vi "Re-Sample Waveform (SubVI).vi"(9 "Filtered w/f":dbl[](array[numeric]), 10 "old dt":dbl, 11 "Re Sample Rate(Hz)":dbl=1000.0 format="%#_13g") -> (2 "Re-sampled w/f":dbl[](array[numeric]), 3 "new dt":dbl)   [LabVIEW 2017]
uses:
  <vilib>/measure/NI_MAPro.lvlib
  <vilib>/measure/maresamp.llb/Resample Waveform (single shot).vi
panel:
  out "error out":errorcluster
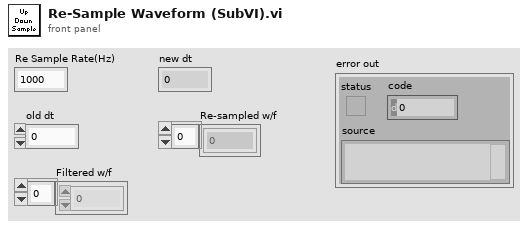
[diagram p1: front panel]
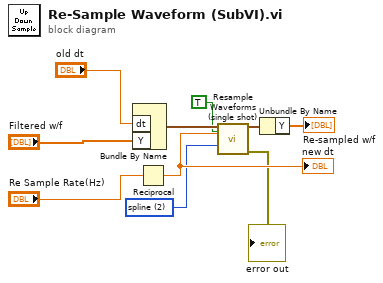
[diagram p0: block diagram]
diagram:
  w4 = u16 2 items=["coerce", "linear", "spline", "FIR filter"] ("interpolation mode")
  n1 = Bundle By Name("dt"="old dt", "Y"="Filtered w/f") -> (w5:waveform(dbl))  [unwired: 1 in]
  n2 = Reciprocal(x="Re Sample Rate(Hz)") -> (1/x=w9:dbl)
  "new dt" <- w9
  n3 = call-poly <vilib>:"Resample Waveforms (single shot).vi"("waveform in"=w5, "open interval? (F)"=TRUE, "dt"=w9, "interpolation mode"=w4) -> ("resampled waveform out"=w6:waveform(dbl), "error out"=→"error out":errorcluster)  [unwired: 8 in, 2 out]
  n4 = Unbundle By Name(w6) -> ("Y"=→"Re-sampled w/f":dbl[])
